vi "Flouish Data Table.vi"() -> ()   [LabVIEW 2020, in "Visualisation.lvclass"]
uses:
  Visualisation.lvclass
  Application/Globals.vi
  <vilib>/Utility/file.llb/Write Delimited Spreadsheet (string).vi
  Data Manager/Data Manager.lvclass
  Application/Application.lvlib
panel:
  in  "Number of days":i32=7
  out "Table Control":string[][](table)
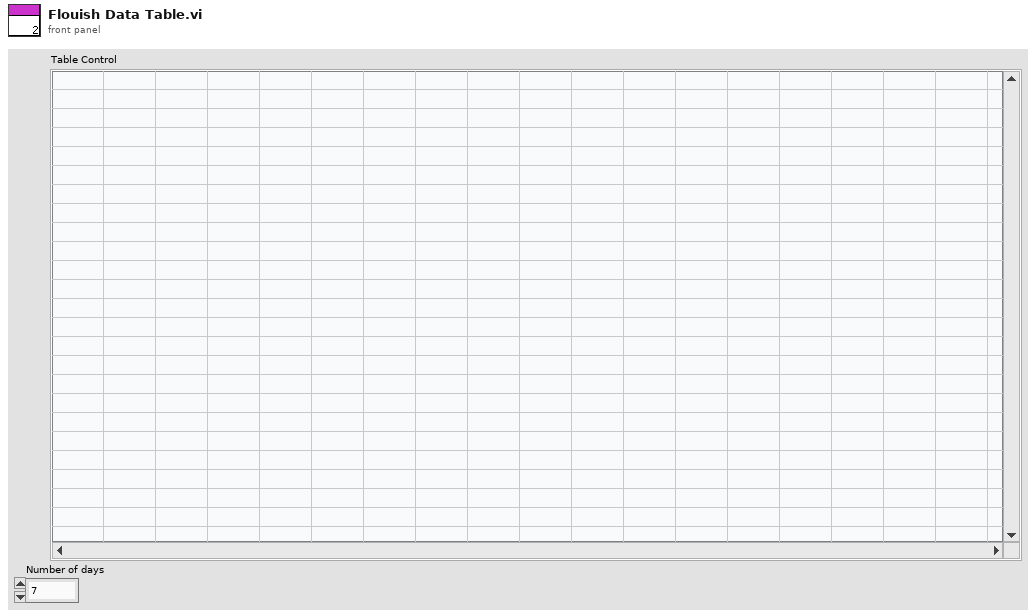
[diagram p1: front panel]
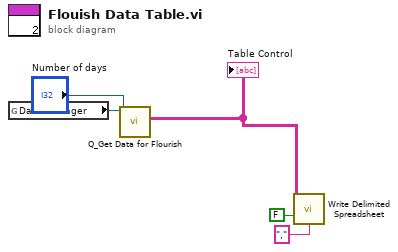
[diagram p0: block diagram]
diagram:
  n1 = global read "Globals.vi" "Data Manager"() -> (w5:refnum<class "Data Manager.lvclass">)
  n2 = call-dynamic "Q_Get Data for Flourish.vi"("Number of days"="Number of days", "Data Manager in"=w5) -> ("Array"=w4:string[][])  [unwired: 7 in, 2 out]
  "Table Control" <- w4
  n3 = call-poly <vilib>:"Write Delimited Spreadsheet.vi"("2D data"=w4, "append to file? (new file:F)"=FALSE, "delimiter (\\t)"="," ("delimiter (\\t)")) -> ()  [unwired: 11 in, 2 out]
